vi "WPI_RelayGetSetRefNum.vi"(8 "error in (no error)":errorcluster, 9 "menu":T1, 10 "refnum name":string, 11 "RelayDevRef":T2={"DevStatus"={"status"=FALSE, "code"=0, "source"=""}, "Relay Channel"=enum."Relay 2", "Relay Direction"=enum."Both directions"}) -> (0 "error out":errorcluster, 2 "names":string[](array[string]), 3 "RelayDevRef":T2={"DevStatus"={"status"=FALSE, "code"=0, "source"=""}, "Relay Channel"=enum."Relay 2", "Relay Direction"=enum."Both directions"})   [LabVIEW 2017]
doc: "Sets a reference into a registry, gets a reference from a registry, or deletes a reference from a registry. The reference is accessed by name, and can be given any unique name.\n\nThis software is licensed. Open the labview\\readme\\WPI Robotics Library Open Source License.txt file for more information."
uses:
  <vilib>/Rock Robotics/WPI/Relay/WPI_RelayDevRef.ctl
  <vilib>/Rock Robotics/SystemInterfaces/DIO/FPGA_DIORelayChannel.ctl
  <vilib>/Rock Robotics/WPI/Relay/WPI_RelayDirection.ctl
  <vilib>/Rock Robotics/WPI/Utilities/Refnum Registry Operation.ctl
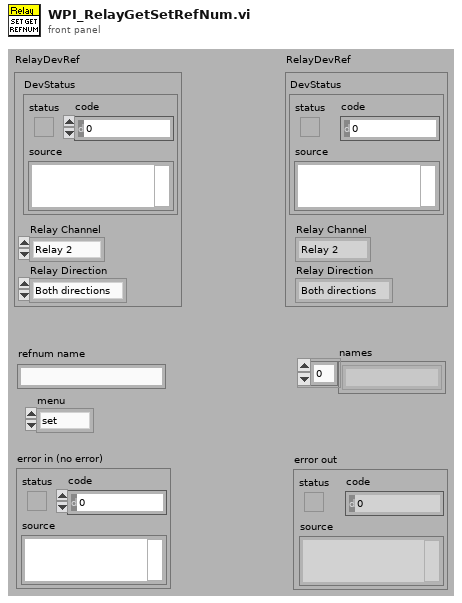
[diagram p1: front panel]
types:
  T1 = typedef "Refnum Registry Operation.ctl" = enum16{"set", "get", "delete", "get all names", "read name"}
  T2 = typedef "WPI_RelayDevRef.ctl" = cluster{"DevStatus":errorcluster, "Relay Channel":T3, "Relay Direction":T4}
  T3 = typedef "FPGA_DIORelayChannel.ctl" = enum8{"Relay 0", "Relay 1", "Relay 2", "Relay 3", "Invalid"}
  T4 = typedef "WPI_RelayDirection.ctl" = enum16{"Both directions", "Forward only", "Reverse only"}
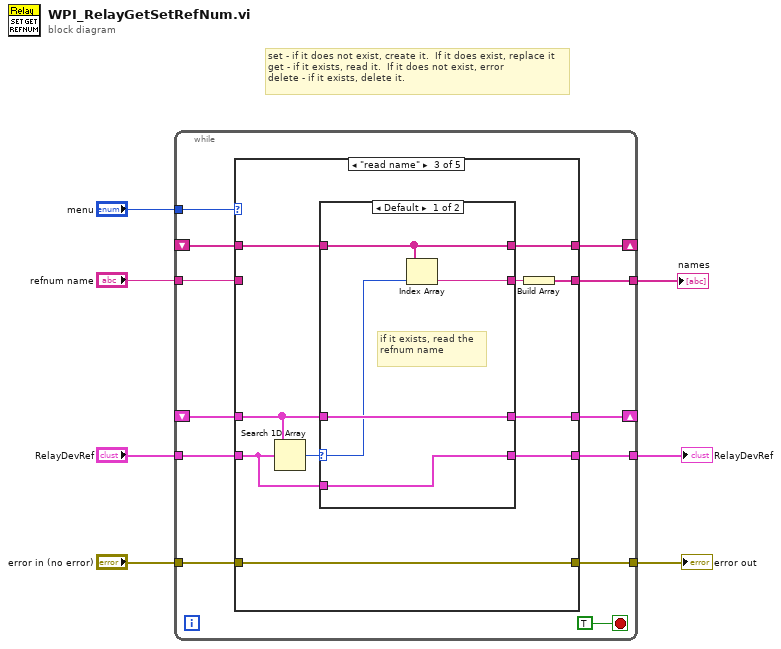
[diagram p0: block diagram]
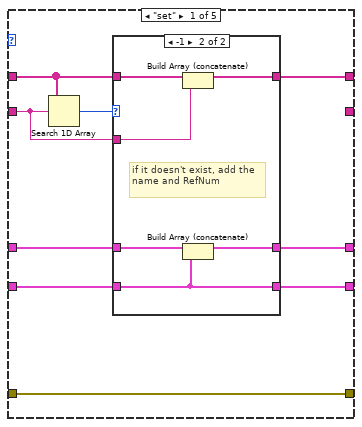
[diagram p2: hidden frame]
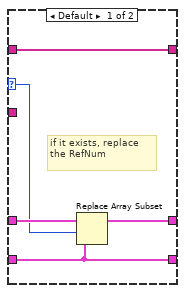
[diagram p3: hidden frame]
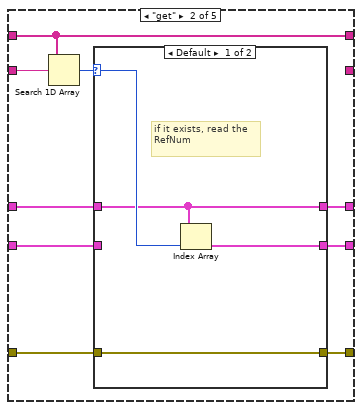
[diagram p4: hidden frame]
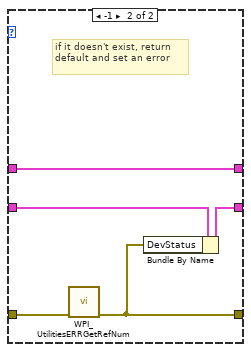
[diagram p5: hidden frame]
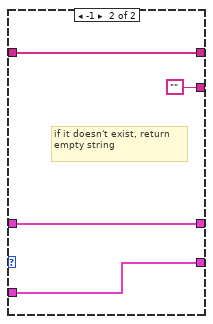
[diagram p6: hidden frame]
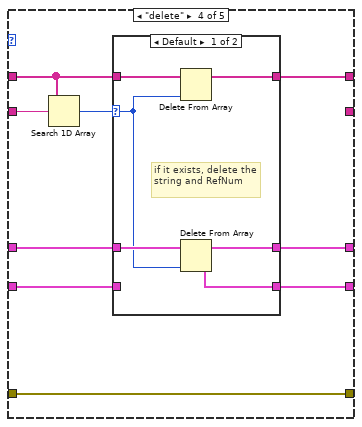
[diagram p7: hidden frame]
diagram:
  # "set - if it does not exist, create it.  If it does exist, replace it\nget - if it exists, read it.  If it does not exist, error\ndelete - if it exists, delete it."
  n1 = while {
    tunnel: "RelayDevRef" -> [w19]
    tunnel: "refnum name" -> [w12]
    tunnel: "error in (no error)" -> [w11]
    shift-right: [w18] -> _
    shift-left: _ -> [w17]
    tunnel: [w16] -> w5
    tunnel: "menu" -> [w15]
    shift-right: [w14] -> _
    shift-left: _ -> [w13]
    tunnel: [w10] -> w3
    tunnel: [w8] -> w1
    stop <- TRUE stop-if-true
    n2 = case shown="\"read name\"" w15 {
      tunnel: w19 -> [w23 w46 w59 w81 w96]
      tunnel: [w22 w45 w67 w80 w97] -> w18
      tunnel: w17 -> [w24 w47 w65 w82 w97]
      tunnel: [w21 w44 w66 w79 w96] -> w16
      tunnel: [w28 w43 w61 w85 w98] -> w14
      tunnel: w13 -> [w27 w43 w62 w84 w98]
      tunnel: w12 -> [w25 w40 _ w77 _]
      tunnel: [w20 w41 w63 w78 w95] -> w10
      tunnel: w11 -> [w20 w42 w63 w78 w95]
      tunnel: [_ _ w58 _ w98] -> w8
      frame "set" {
        n3 = Search 1D Array(1D array=w27, element=w25) -> (index of element=w26:i32)  [unwired: 1 out]
        n4 = case shown="-1" w26 {
          selector: w26 -> [w31 _]
          tunnel: [w33 w39] -> w28
          tunnel: w27 -> [w33 w38]
          tunnel: w25 -> [_ w34]
          tunnel: w24 -> [w32 w37]
          tunnel: w23 -> [w29 w35]
          tunnel: [w30 w36] -> w22
          tunnel: [w29 w35] -> w21
          frame Default {
            # "if it exists, replace the RefNum"
            n5 = Replace Array Subset(array=w32, new element=w29, index=w31) -> (w30:T2[])
          }
          frame -1 {
            # "if it doesn't exist, add the name and RefNum"
            n6 = Build Array (concatenate)(w38, w34) -> (w39:string[])
            n7 = Build Array (concatenate)(w37, w35) -> (w36:T2[])
          }
        }
      }
      frame "get" {
        n8 = Search 1D Array(1D array=w43, element=w40) -> (index of element=w48:i32)  [unwired: 1 out]
        n9 = case shown="Default" w48 {
          selector: w48 -> [w52 _]
          tunnel: w47 -> [w50 w57]
          tunnel: w46 -> [_ w55]
          tunnel: [w50 w57] -> w45
          tunnel: [w51 w54] -> w44
          tunnel: w42 -> [w49 w56]
          tunnel: [w49 w53] -> w41
          frame Default {
            # "if it exists, read the RefNum"
            n10 = Index Array(array=w50, index=w52) -> (element=w51:T2)
          }
          frame -1 {
            # "if it doesn't exist, return default and set an error"
            n11 = call <vilib>:"WPI_UtilitiesERRGetRefNum.vi"("error in (no error)"=w56) -> ("ERRGetRefNum"=w53:errorcluster)  [unwired: 10 out]
            n12 = Bundle By Name(cluster=w55, "DevStatus"=w53) -> (w54:T2)
          }
        }
      }
      frame "read name" {
        n13 = Search 1D Array(1D array=w65, element=w59) -> (index of element=w64:i32)  [unwired: 1 out]
        n14 = case shown="Default" w64 {
          selector: w64 -> [w69 _]
          tunnel: w65 -> [w72 w76]
          tunnel: [w72 w76] -> w67
          tunnel: [w68 w75] -> w66
          tunnel: w62 -> [w70 w74]
          tunnel: [w70 w74] -> w61
          tunnel: [w71 ""] -> w60
          tunnel: w59 -> [w68 w75]
          frame Default {
            # "if it exists, read the refnum name"
            n15 = Index Array(array=w70, index=w69) -> (element=w71:string)
          }
          frame -1 {
            # "if it doesn't exist, return empty string"
          }
        }
        n16 = Build Array(w60) -> (w58:string[])
      }
      frame "delete" {
        n17 = Search 1D Array(1D array=w84, element=w77) -> (index of element=w83:i32)  [unwired: 1 out]
        n18 = case shown="Default" w83 {
          selector: w83 -> [w86 _]
          tunnel: [w87 w93] -> w85
          tunnel: w84 -> [w88 w93]
          tunnel: w82 -> [w91 w92]
          tunnel: w81 -> [_ w94]
          tunnel: [w90 w92] -> w80
          tunnel: [w89 w94] -> w79
          frame Default {
            # "if it exists, delete the string and RefNum"
            n19 = Delete From Array(array=w88, index=w86) -> (array with subset deleted=w87:string[])  [unwired: 1 in, 1 out]
            n20 = Delete From Array(array=w91, index=w86) -> (deleted portion=w89:T2, array with subset deleted=w90:T2[])  [unwired: 1 in]
          }
          frame -1 {
            # "if it doesn't exist, do nothing"
          }
        }
      }
      frame "get all names", Default {
      }
    }
  }
  "error out" <- w3
  "RelayDevRef" <- w5
  "names" <- w1
